vi "Configure Ramp Symmetry.vi"(8 "error in (no error)":errorcluster, 9 "Ramp Symmetry (50.00 %)":dbl=50.0 min=0.0 max=100.0 step=1.0 format="%.2f", 10 "Channel (0: Channel 1)":u16(ring) items=["Channel 1", "Channel 2"], 11 "VISA resource name":refnum<visa-resource-name>) -> (0 "error out":errorcluster, 3 "VISA resource name out":refnum<visa-resource-name>)   [LabVIEW 2013, in "AWG.lvlib" / "Tektronix AFG 3000 Series.lvlib"]
doc: "Configures the ramp symmetry for Ramp waveforms."
uses:
  Tektronix AFG 3000 Series.lvlib
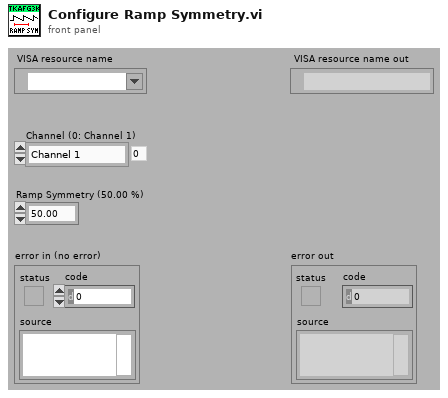
[diagram p1: front panel]
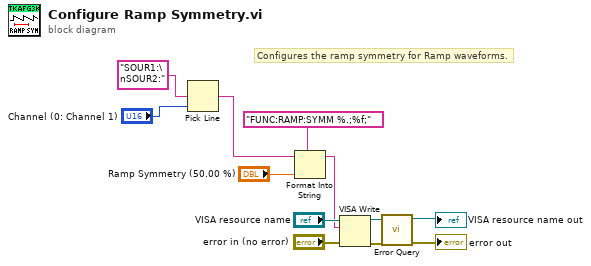
[diagram p0: block diagram]
diagram:
  # "Configures the ramp symmetry for Ramp waveforms."
  n1 = Pick Line(multi-line string="SOUR1:\nSOUR2:" ("string (\"\")"), line index="Channel (0: Channel 1)") -> (output string=w1:string)  [unwired: 1 in]
  n2 = Format Into String(format string="FUNC:RAMP:SYMM %.;%f;", initial string=w1, "Ramp Symmetry (50.00 %)") -> (resulting string=w4:string)  [unwired: 1 in, 1 out]
  n3 = VISA Write(VISA resource name="VISA resource name", write buffer=w4, error in (no error)="error in (no error)") -> (VISA resource name out=w10:refnum<visa-resource-name>, error out=w11:errorcluster)  [unwired: 1 out]
  n4 = call "Error Query.vi"("error in (no error)"=w11, "VISA resource name"=w10) -> ("error out"=→"error out":errorcluster, "VISA resource name out"=→"VISA resource name out":refnum<visa-resource-name>)  [unwired: 6 in, 2 out]
